vi "Read Normal Measure Item.vi"(0 "VISA resource name":refnum<visa-resource-name>, 1 "Element (1: Element 1)":u16(ring)=1 items=["", "Element1", "Element2", "Element3", "Sigma"], 5 "Measure Item (0: V)":u16(ring) items=["V", "A", "W", "VA", "var", "PF", "deg", "V Hz", "A Hz", "Wh", "Wh+", "Wh-", "Ah", "Ah+", "Ah-", "Vpk", "Apk", "Math"], 11 "error in (no error)":errorcluster) -> (4 "VISA resource name out":refnum<visa-resource-name>, 6 "Measure Value":sgl format="%^.3e", 15 "error out":errorcluster)   [LabVIEW 2011, in "Yokogawa WT200 Series.lvlib"]
doc: "This VI reads measurement value of the specified item from the WT200 Series."
uses:
  G:/Engineering/Retail/LabV/instr.lib/Yokogawa WT200 Series/Yokogawa WT200 Series.lvlib
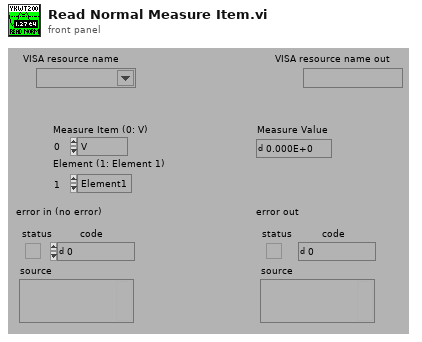
[diagram p1: front panel]
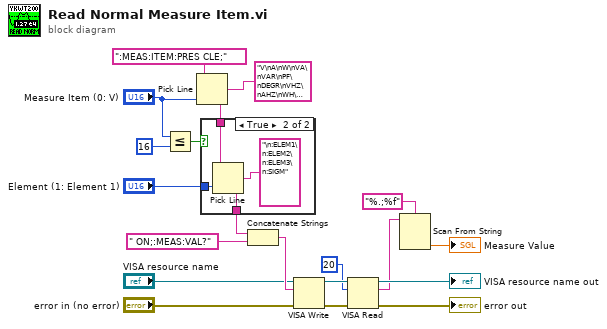
[diagram p0: block diagram]
diagram:
  n1 = Less Or Equal?(x="Measure Item (0: V)", y=u16 16) -> (x <= y?=w7:bool)
  n2 = Pick Line(string ("")=":MEAS:ITEM:PRES CLE;", multi-line string="V\nA\nW\nVA\nVAR\nPF\nDEGR\nVHZ\nAHZ\nWH\nWHP\nWHM\nAH\nAHP\nAHM\nVPK\nAPK\nMATH", line index="Measure Item (0: V)") -> (output string=w4:string)
  n3 = case shown="True" w7 {
    tunnel: w4 -> [w21 w24]
    tunnel: [w21 w23] -> w3
    tunnel: "Element (1: Element 1)" -> [_ w22]
    frame False {
      # "Time or Math"
    }
    frame True {
      n4 = Pick Line(string ("")=w24, multi-line string="\n:ELEM1\n:ELEM2\n:ELEM3\n:SIGM", line index=w22) -> (output string=w23:string)
    }
  }
  n5 = Concatenate Strings(w3, " ON;:MEAS:VAL?") -> (w19:string)
  n6 = VISA Write(VISA resource name="VISA resource name", write buffer=w19, error in (no error)="error in (no error)") -> (VISA resource name out=w16:refnum<visa-resource-name>, error out=w17:errorcluster)  [unwired: 1 out]
  n7 = VISA Read(VISA resource name=w16, byte count=u32 20, error in (no error)=w17) -> (VISA resource name out=→"VISA resource name out":refnum<visa-resource-name>, read buffer=w12:string, error out=→"error out":errorcluster)  [unwired: 1 out]
  n8 = Scan From String(format string="%.;%f", input string=w12) -> (output 1=→"Measure Value":sgl)  [unwired: 3 in, 3 out]
